vi "SaveToText.vi"(5 "Text.Selection":T1, 8 "error in (no error)":errorcluster, 9 "Additional Header":string, 10 "editor refs":refnum<vi>[](array[refnum]), 11 "Tree ref":refnum<vi>) -> (0 "error out":errorcluster, 1 "String":string)   [LabVIEW 2020, in "ScriptManager.lvlib"]
uses:
  ScriptManager.lvlib
  <vilib>/Utility/miscctls.llb/LVSelectionTypeDef.ctl
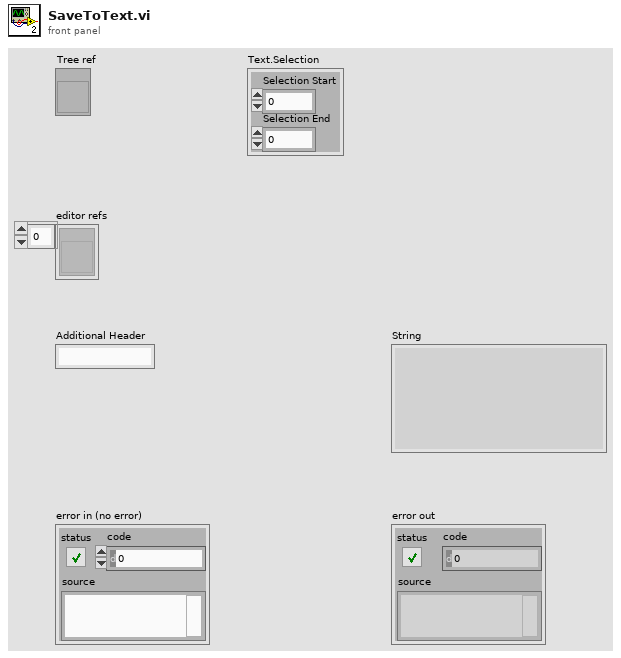
[diagram p1: front panel]
types:
  T1 = typedef "LVSelectionTypeDef.ctl" = cluster{"Selection Start":u32, "Selection End":u32}
  T2 = cluster{"[0]":string, "[1]":string, "[2]":string, "[3]":string, "[4]":string}
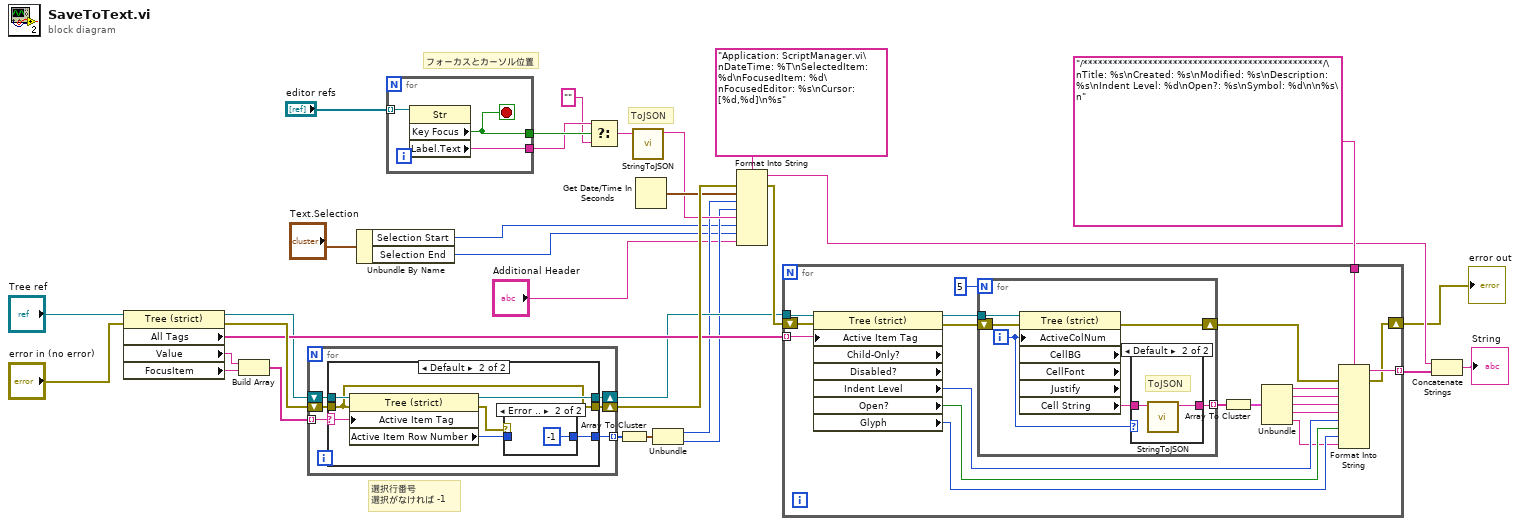
[diagram p0: block diagram]
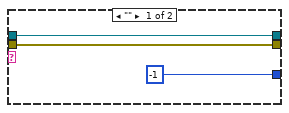
[diagram p2: hidden frame]
diagram:
  # "フォーカスとカーソル位置"
  # "ToJSON"
  # "選択行番号\n選択がなければ -1"
  n1 = property class="Tree (strict)"(reference="Tree ref", error in="error in (no error)") -> (reference out=w18:refnum<vi>, error out=w27:errorcluster, "All Tags"=w19:string[], "Value"=w16:string, "FocusItem"=w8:string)
  n2 = Build Array(w16, w8) -> (w9:string[])
  n3 = for {
    tunnel: [w37] -> w25 mode=indexing
    tunnel: w9 -> [w33] mode=indexing
    shift-right: [w36] -> w22
    shift-left: w27 -> [w38]
    shift-right: [w34] -> w17
    shift-left: w18 -> [w35]
    n4 = case shown="Default" w33 {
      selector: w33 -> [_ w46]
      tunnel: w38 -> [w39 w42]
      tunnel: [-1 ("Active Item Row Number") w44] -> w37
      tunnel: [w39 w42] -> w36
      tunnel: w35 -> [w40 w48]
      tunnel: [w40 w47] -> w34
      frame "" {
      }
      frame Default {
        n5 = property class="Tree (strict)"(reference=w48, error in=w42, "Active Item Tag"=w46) -> (reference out=w47:refnum<vi>, error out=w43:errorcluster, "Active Item Row Number"=w45:i32)
        n6 = case shown="Error .." w43 {
          tunnel: w45 -> [w49 _]
          tunnel: [w49 -1 ("Active Item Row Number")] -> w44
          frame No Error {
          }
          frame Error {
          }
        }
      }
    }
  }
  n7 = Unbundle By Name("Text.Selection") -> ("Selection Start"=w3:u32, "Selection End"=w2:u32)
  n8 = for {
    tunnel: "editor refs" -> [w53] mode=indexing
    tunnel: [w52] -> w13
    tunnel: [w51] -> w14
    stop <- w51 stop-if-true
    n9 = property class="Str"(reference=w53) -> ("Key Focus"=w51:bool, "Label.Text"=w52:string)  [unwired: 1 in, 2 out]
  }
  n10 = Select(t=w13, s=w14, f="") -> (s? t:f=w11:string)
  n11 = Array To Cluster(array=w25) -> (cluster=w7:cluster{"[0]":i32, "[1]":i32})
  n12 = call "StringToJSON.vi"("input text"=w11) -> ("JSON string"=w10:string)  [unwired: 10 in]
  n13 = Get Date/Time In Seconds() -> (seconds since 1Jan1904=w15:timestamp)
  n14 = Unbundle(w7) -> ("[0]"=w6:i32, "[1]"=w5:i32)
  n15 = Format Into String(format string="Application: ScriptManager.vi\nDateTime: %T\nSelectedItem: %d\nFocusedItem: %d\nFocusedEditor: %s\nCursor: [%d,%d]\n%s", error in=w22, w15, w6, w5, w10, w3, w2, "Additional Header") -> (resulting string=w24:string, error out=w21:errorcluster)  [unwired: 1 in]
  n16 = for {
    tunnel: w19 -> [w72] mode=indexing
    tunnel: w17 -> [w73]
    tunnel: "/************************************************/\nTitle: %s\nCreated: %s\nModified: %s\nDescription: %s\nIndent Level: %d\nOpen?: %s\nSymbol: %d\n\n%s\n" ("format string") -> [w67]
    tunnel: [w59] -> w30 mode=indexing
    shift-right: [w54] -> w20
    shift-left: w21 -> [w57]
    n17 = property class="Tree (strict)" props=["Active Item Tag", "Child-Only?", "Disabled?", "Indent Level", "Open?", "Glyph"](reference=w73, error in=w57, "Active Item Tag"=w72) -> (reference out=w71:refnum<vi>, error out=w56:errorcluster, "Indent Level"=w62:i32, "Open?"=w61:bool, "Glyph"=w60:i32)  [unwired: 2 out]
    n18 = for {
      N: 5 -> [_]
      tunnel: w71 -> [w79]
      tunnel: [w77] -> w69 mode=indexing
      shift-right: [w74] -> w55
      shift-left: w56 -> [w75]
      i -> [w76]
      n19 = property class="Tree (strict)" props=["ActiveColNum", "CellBG", "CellFont", "Justify", "Cell String"](reference=w79, error in=w75, "ActiveColNum"=w76) -> (error out=w74:errorcluster, "Cell String"=w78:string)  [unwired: 4 out]
      n20 = case shown="Default" w76 {
        tunnel: w78 -> [w80 w82]
        tunnel: [w80 w81] -> w77
        frame 4 {
        }
        frame Default {
          # "ToJSON"
          n21 = call "StringToJSON.vi"("input text"=w82) -> ("JSON string"=w81:string)  [unwired: 10 in]
        }
      }
    }
    n22 = Array To Cluster(array=w69) -> (cluster=w68:T2)
    n23 = Unbundle(w68) -> ("[0]"=w66:string, "[1]"=w65:string, "[2]"=w64:string, "[3]"=w63:string, "[4]"=w58:string)
    n24 = Format Into String(format string=w67, error in=w55, w66, w65, w64, w63, w62, w61, w60, w58) -> (resulting string=w59:string, error out=w54:errorcluster)  [unwired: 1 in]
  }
  "error out" <- w20
  n25 = Concatenate Strings(w24, w30) -> (→"String":string)
